vi "Periodic Tasks.vi"(8 "error in":errorcluster) -> ()   [LabVIEW 2019]
doc: "This VI runs in parallel to other tasks. It can contain as many user-defined periodic loops as you need. These can carry out PID or other sorts of timed response."
uses:
  <vilib>/Rock Robotics/WPI/ThirdParty/Phoenix-LabVIEW/Motor Controller/Controls/CTRE_Phoenix_MotorControl_ControlMode.ctl
  Control 1.ctl
  <vilib>/Rock Robotics/WPI/Solenoid/WPI_SolenoidValue.ctl
  <vilib>/Rock Robotics/WPI/ThirdParty/Phoenix-LabVIEW/Motor Controller/Get/CTRE_Phoenix_MotorController_GetSelectedSensorData.vi
  <vilib>/Rock Robotics/WPI/ThirdParty/Phoenix-LabVIEW/Motor Controller/Get/CTRE_Phoenix_MotorController_IntegratedSensorData_TalonFX.vi
  <vilib>/Rock Robotics/WPI/ThirdParty/Phoenix-LabVIEW/Motor Controller/Get/CTRE_Phoenix_MotorController_GetLimitSwitchStates.vi
  <vilib>/Rock Robotics/WPI/Solenoid/WPI_SolenoidSetEnum.vi
  <vilib>/Rock Robotics/WPI/RobotDrive/WPI_RobotDriveArcadeDrive_Standard(NoSaturation).vi
  <vilib>/Rock Robotics/WPI/ThirdParty/Phoenix-LabVIEW/Motor Controller/Get/CTRE_Phoenix_MotorController_GetQuadratureData.vi
  Talon SRX State Machine Enum.ctl
panel:
  in  "D":dbl
  in  "I":dbl
  in  "P":dbl=1.5
  in  "D 6":dbl
  in  "I 6":dbl
  in  "P 6":dbl=1.6
  in  "D 5":dbl
  in  "I 5":dbl
  in  "P 5":dbl=1.6
  out "Chicken 500 Low Home":bool
  out "Position":dbl format="%.2f"
  out "Dial":dbl(knob)=26.0 scale=26.0..156.0
  out "Degrees":dbl
  in  "D 2":dbl
  in  "I 2":dbl
  in  "P 2":dbl=1.6
  out "Low Home":bool
  out "Quadrature Position 2":i32
  # "90"
  # "45"
  # "F 90"
  # "F 45"
  # "Home"
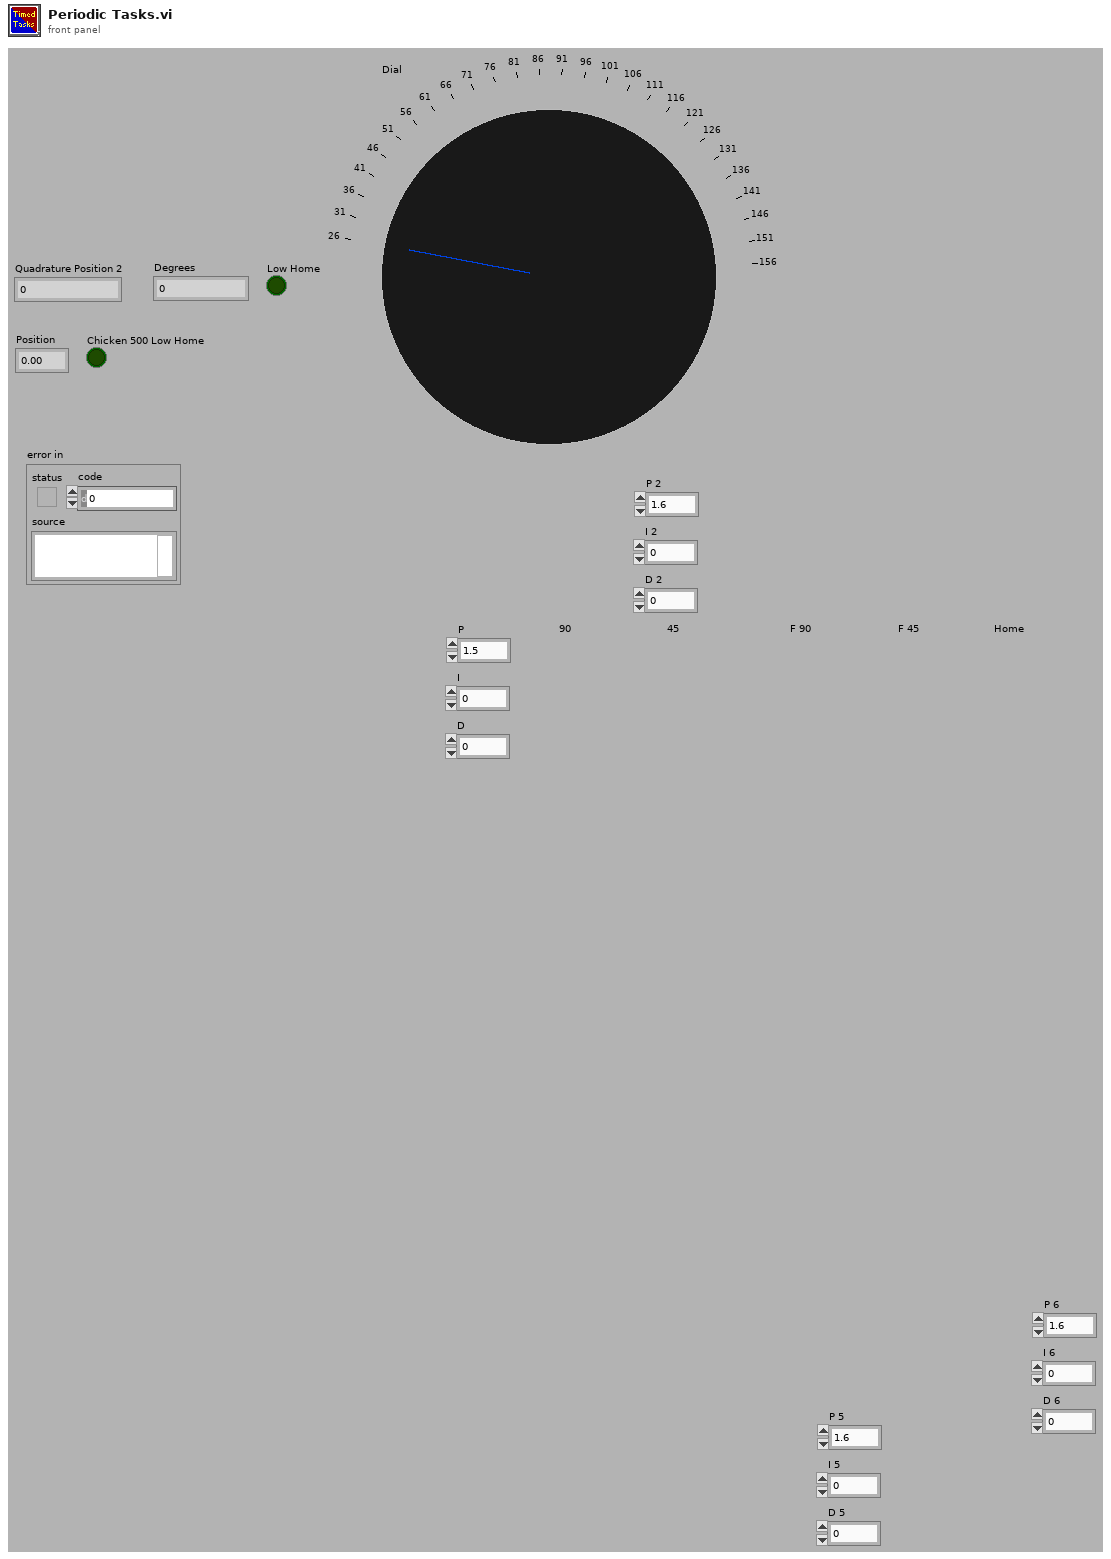
[diagram p1: front panel]
types:
  T1 = typedef "Talon SRX State Machine Enum.ctl" = enum16{"Wait", "Move 0", "Move 1", "Move 2", "Init"}
  T2 = typedef "Control 1.ctl" = enum16{"Wait", "F Move 0", "F Move 1", "F Move 2"}
  T3 = typedef "WPI_JoystickDevRef.ctl" = cluster{"Device":T4}
  T4 = typedef "WPI_JoystickDeviceEnum.ctl" = enum16{"USB 0", "USB 1", "USB 2", "USB 3", "USB 4", "USB 5"}
  T5 = typedef "WPI_MotorControlDeviceRef.ctl" = cluster{"DeviceStatus":errorcluster, "Type":T6, "PWM":cluster{"PWM Channel":T7, "DeadBand":T8}, "CAN":cluster{"Device Number":u8, "SetOutput VI Ref":variant, "GetOutput VI Ref":variant, "Enable VI Ref":variant, "Disable VI Ref":variant, "Data":variant}, "Invert":bool, "DIO PWM":cluster{"PWM \"Enable\" Channel":T7, "DIOChannel":T9, "PWM Rate":dbl}}
  T6 = typedef "WPI_MotorControlType.ctl" = enum16{"PWM", "CAN", "DIO PWM"}
  T7 = typedef "FPGA_DIOPWMChannel.ctl" = enum8{"PWM 0", "PWM 1", "PWM 2", "PWM 3", "PWM 4", "PWM 5", "PWM 6", "PWM 7", "PWM 8", "PWM 9", "PWM MXP 0", "PWM MXP 1", "PWM MXP 2", "PWM MXP 3", "PWM MXP 4", "PWM MXP 5", "PWM MXP 6", "PWM MXP 7", "PWM MXP 8", "PWM MXP 9", "Invalid"}
  T8 = typedef "WPI_PWMDeadband.ctl" = cluster{"Name":string, "maxPositivePwm":i32, "minPositivePwm":i32, "centerPwm":i32, "maxNegativePwm":i32, "minNegativePwm":i32, "angularRange":u16}
  T9 = typedef "FPGA_DIOChannel.ctl" = enum8{"DIO 0", "DIO 1", "DIO 2", "DIO 3", "DIO 4", "DIO 5", "DIO 6", "DIO 7", "DIO 8", "DIO 9", "DIO MXP 0", "DIO MXP 1", "DIO MXP 2", "DIO MXP 3", "DIO MXP 4", "DIO MXP 5", "DIO MXP 6", "DIO MXP 7", "DIO MXP 8", "DIO MXP 9", "DIO MXP 10", "DIO MXP 11", "DIO MXP 12", "DIO MXP 13", "DIO MXP 14", "DIO MXP 15", "SPI Port CS1", "SPI Port CS2", "SPI Port CS3", "SPI Port MISO", "SPI Port MOSI", "Invalid"}
  T10 = typedef "CTRE_Phoenix_MotorControl_ControlMode.ctl" = u16
  T11 = typedef "WPI_DigitalInputDevRef.ctl" = cluster{"DevStatus":errorcluster, "DIO Channel":T9}
  T12 = typedef "WPI_SolenoidValue.ctl" = enum16{"Off", "On", "Forward", "Reverse"}
  T13 = typedef "WPI_RobotDriveDevRef.ctl" = cluster{"DevStatus":errorcluster, "Motors[]":T5[], "Square Inputs":bool, "Max Output":dbl}
  T14 = typedef "WPI_SolenoidDevRef.ctl" = cluster{"DevStatus":errorcluster, "Pneumatics Control Module":u8, "Forward Solenoid Channel":T15, "Reverse Solenoid Channel":T15}
  T15 = typedef "WPI_SolenoidChannel.ctl" = enum8{"Solenoid 0", "Solenoid 1", "Solenoid 2", "Solenoid 3", "Solenoid 4", "Solenoid 5", "Solenoid 6", "Solenoid 7", "Invalid"}
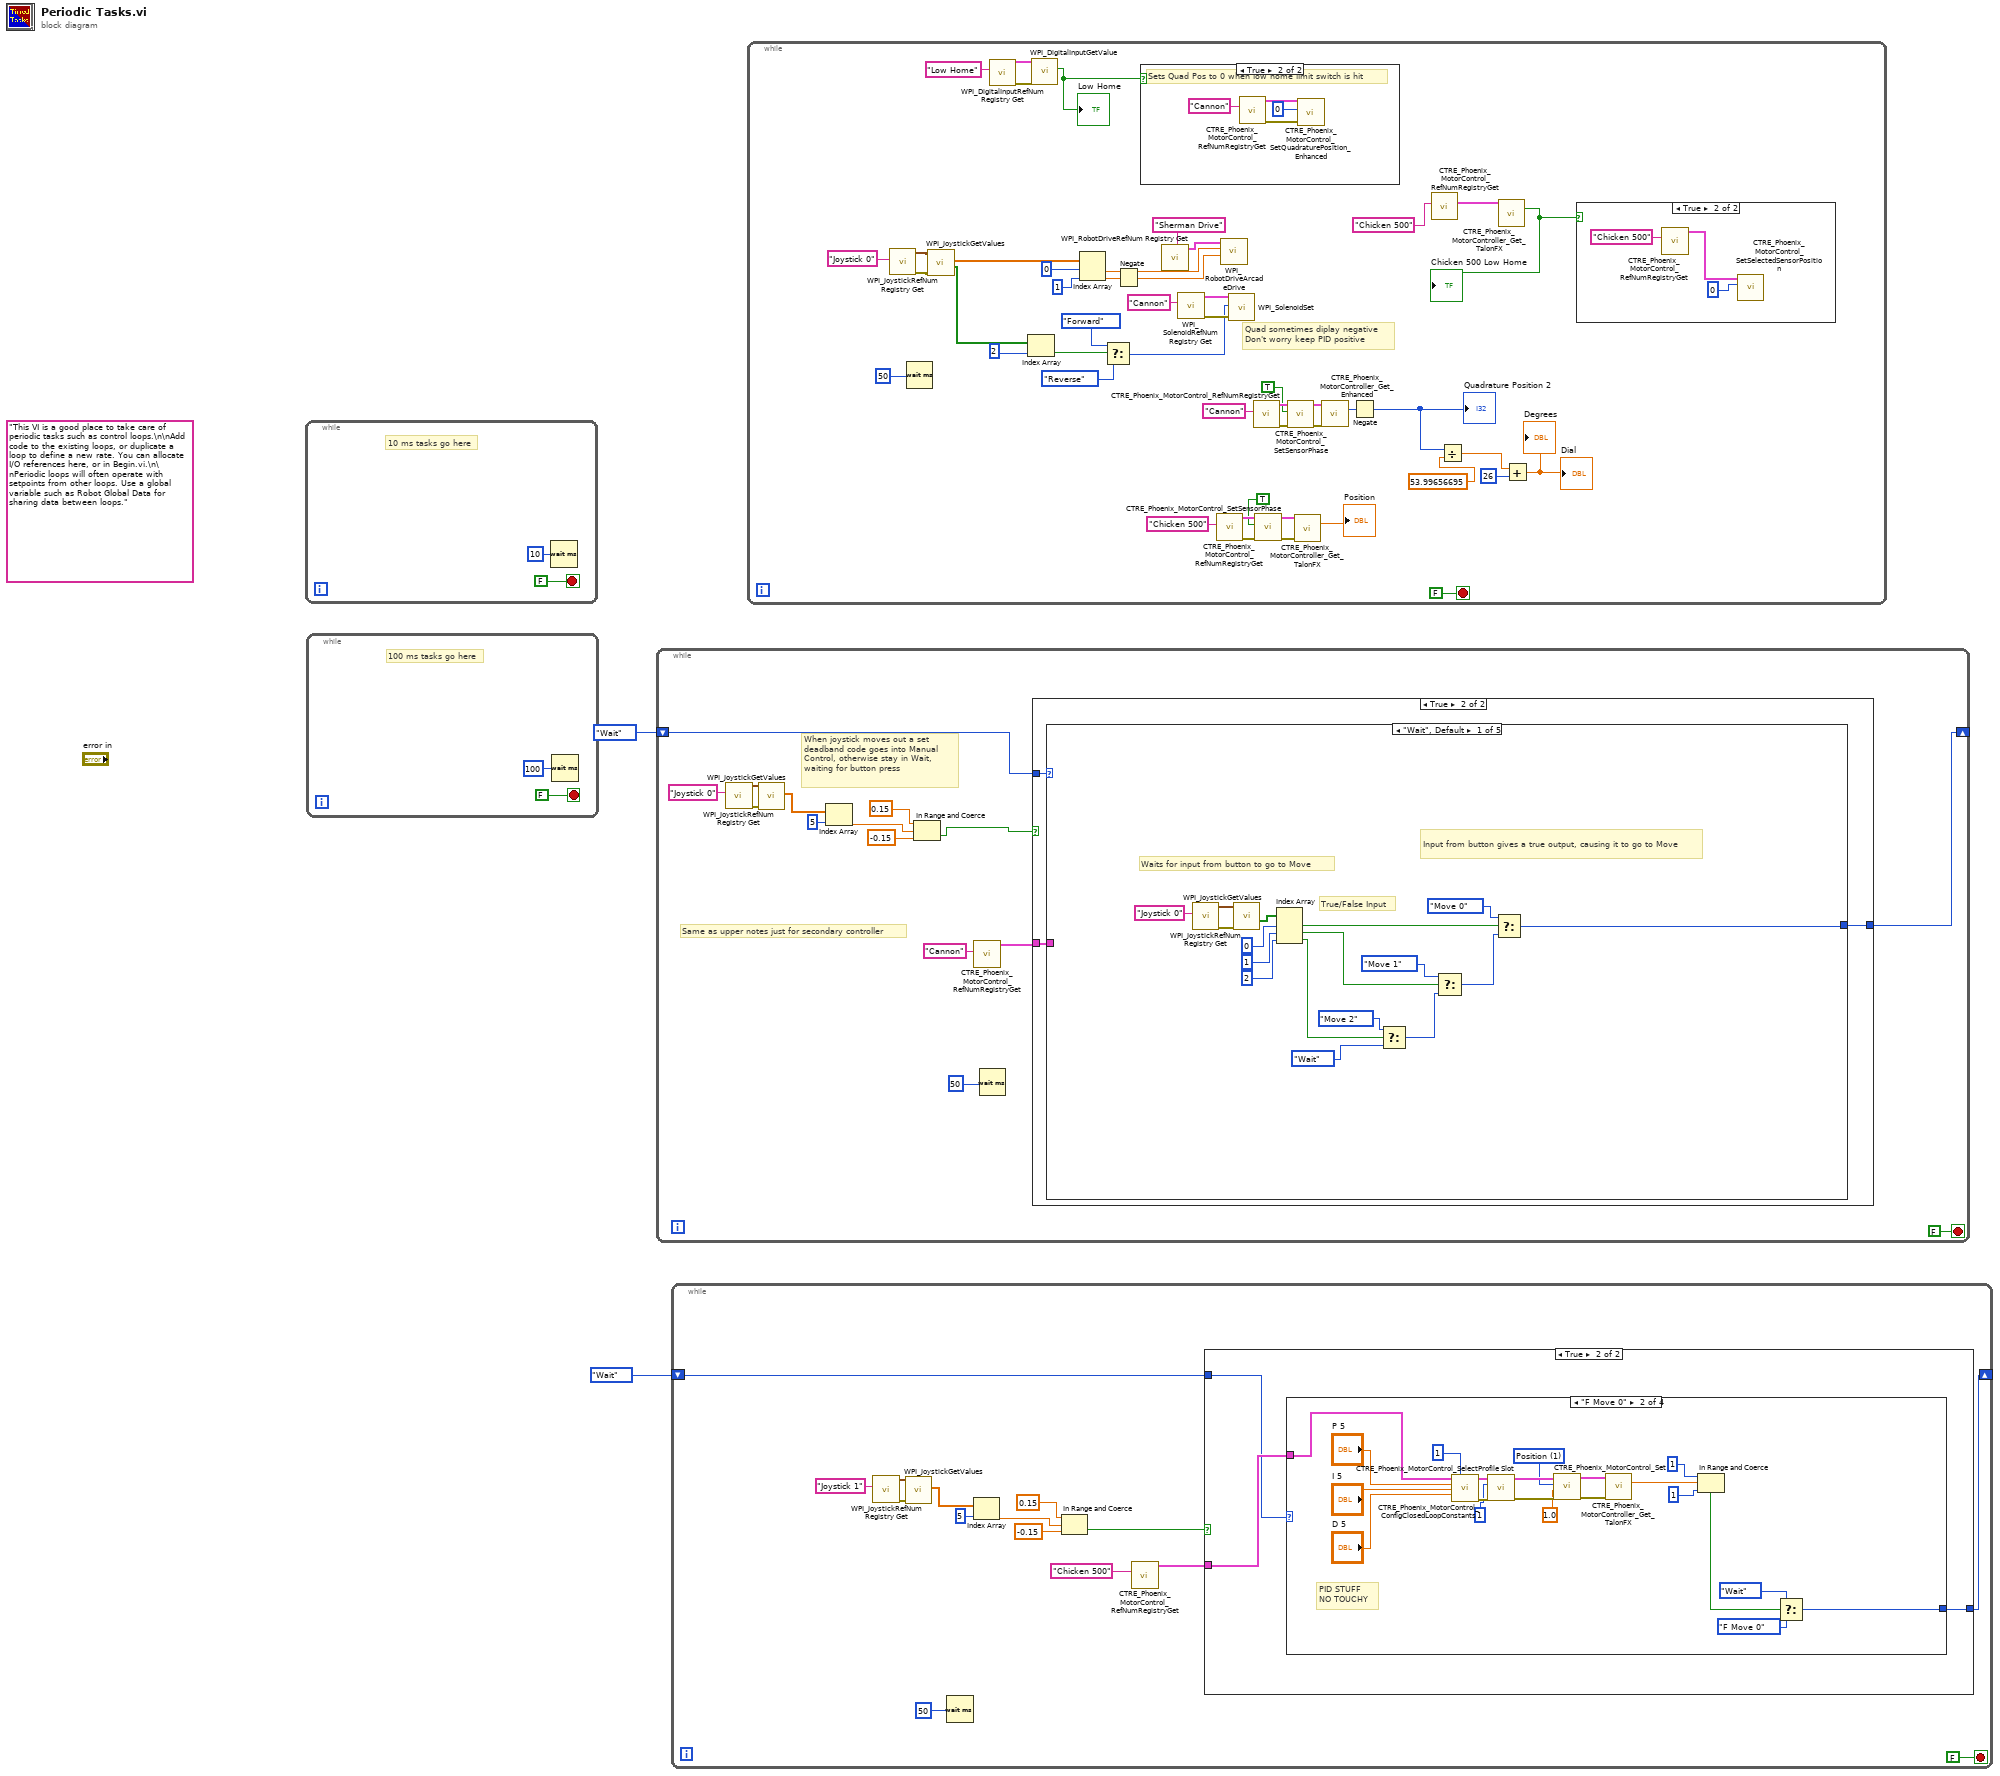
[diagram p0: block diagram]
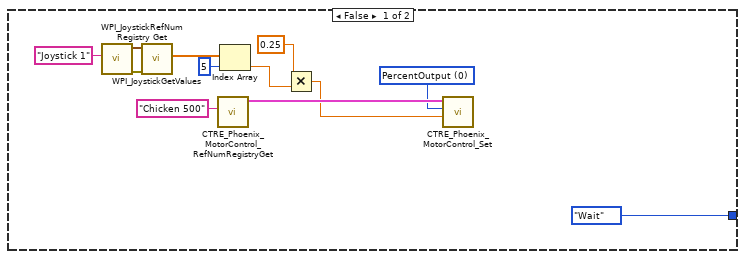
[diagram p2: hidden frame]
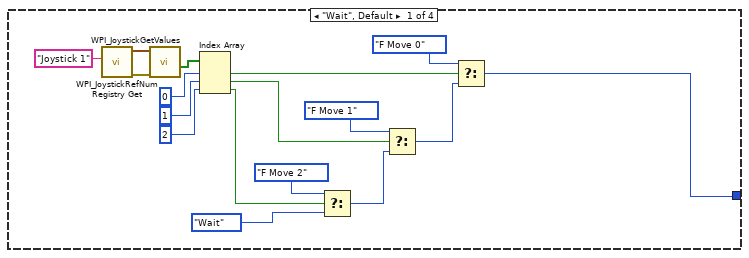
[diagram p3: hidden frame]
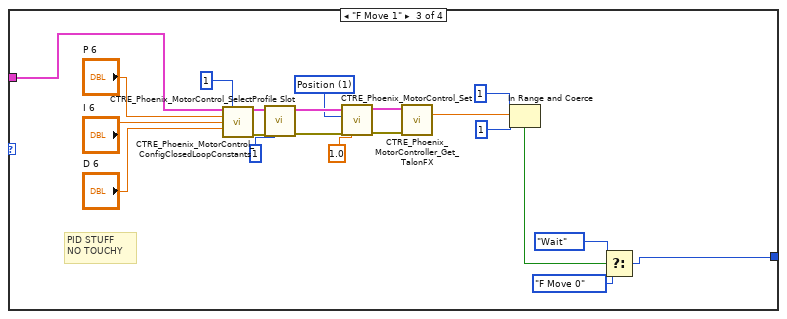
[diagram p4: hidden frame]
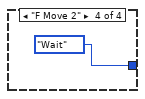
[diagram p5: hidden frame]
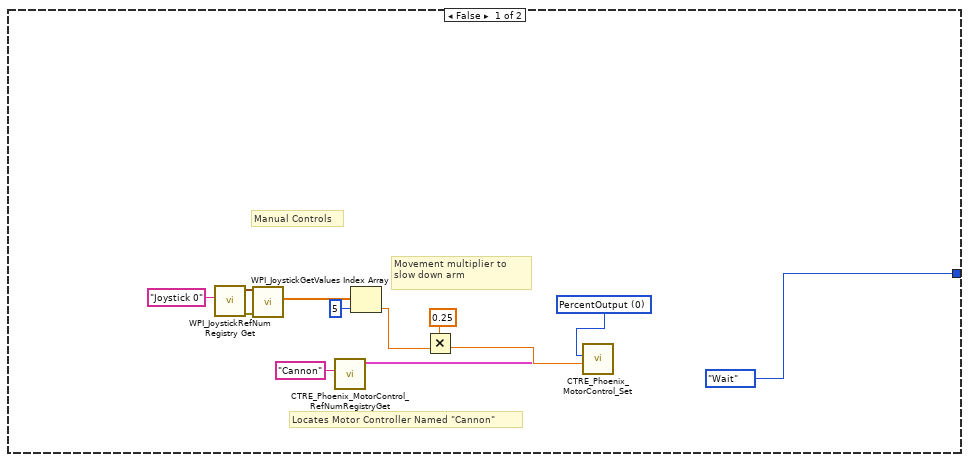
[diagram p8: hidden frame]
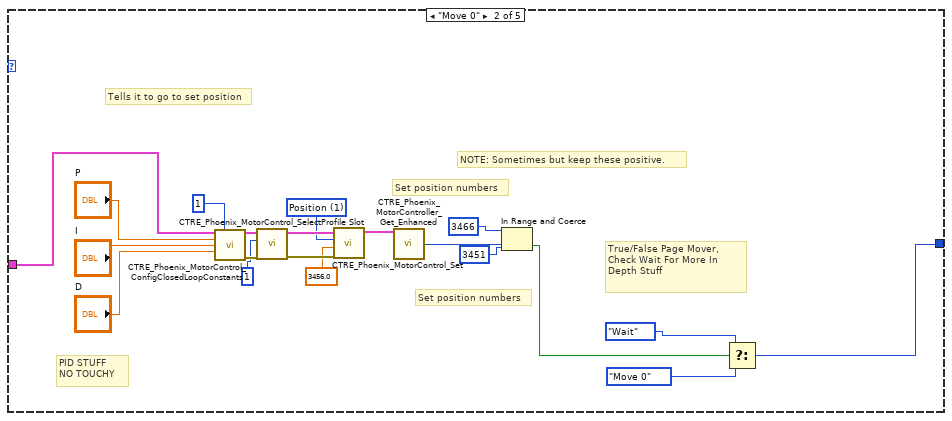
[diagram p9: hidden frame]
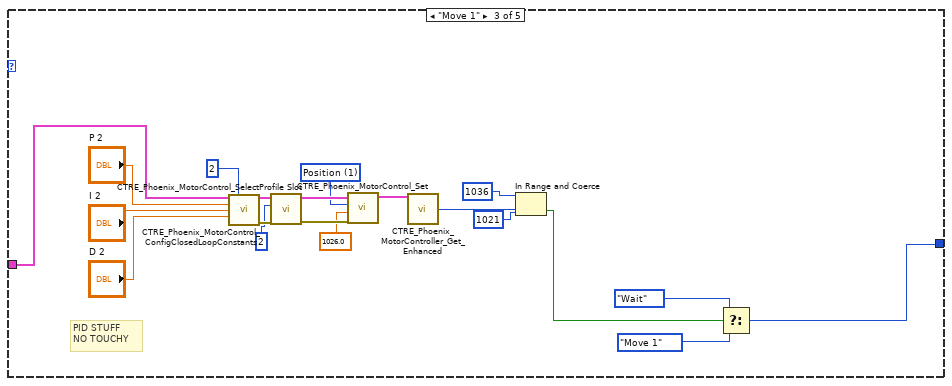
[diagram p10: hidden frame]
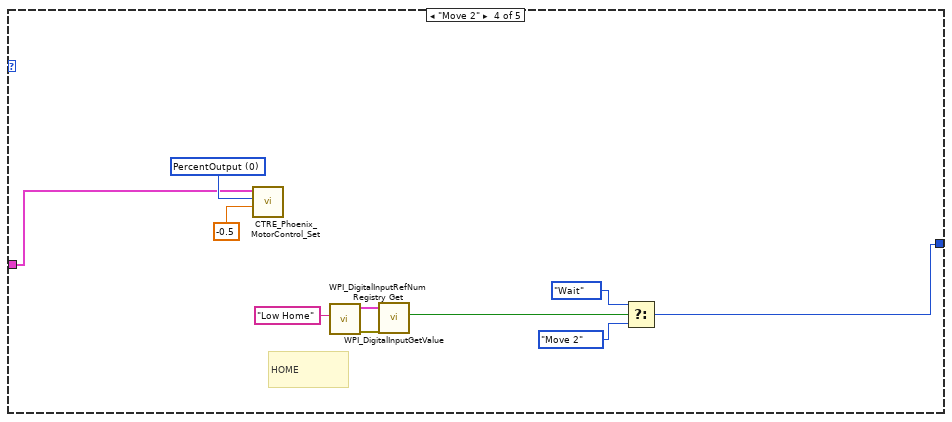
[diagram p11: hidden frame]
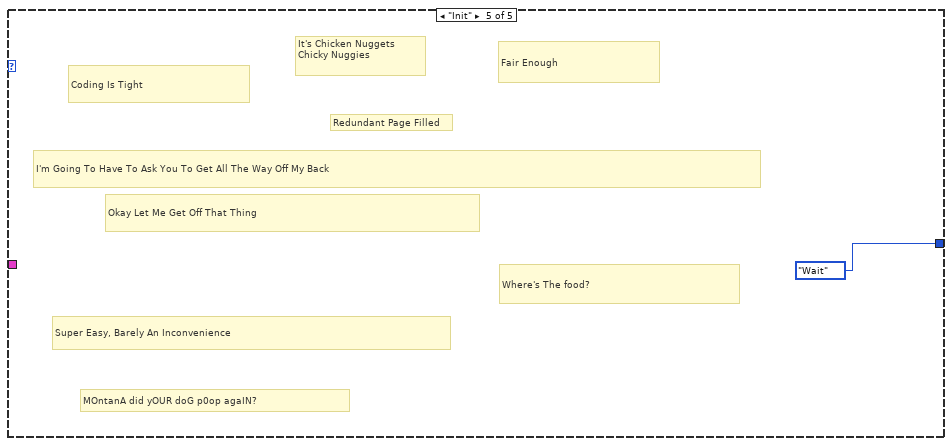
[diagram p12: hidden frame]
diagram:
  (unwired) "This VI is a good place to take care of periodic tasks such as control loops.\n\nAdd code to the existing loops, or duplicate a loop to define a new rate. You can allocate I/O references here, or in Begin.vi.\n\nPeriodic loops will often operate with setpoints from other loops. Use a global variable such as Robot Global Data for sharing data between loops."
  n1 = while {
    stop <- FALSE stop-if-true
    # "10 ms tasks go here"
    n2 = Wait (ms)(milliseconds to wait=u32 10) -> ()  [unwired: 1 out]
  }
  n3 = while {
    stop <- FALSE stop-if-true
    # "100 ms tasks go here"
    n4 = Wait (ms)(milliseconds to wait=u32 100) -> ()  [unwired: 1 out]
  }
  n5 = while {
    shift-right: [w7] -> _
    shift-left: Talon_SRX_State_Machine_Enum."Wait" -> [w21]
    stop <- FALSE stop-if-true
    # "Same as upper notes just for secondary controller"
    # "When joystick moves out a set deadband code goes into Manual Control, otherwise stay in Wait, waiting for button press"
    n6 = call <vilib>:"WPI_JoystickRefNum Registry Get.vi"("refnum name"="Joystick 0") -> ("error out"=w19:errorcluster, "JoystickDevRef"=w11:T3)  [unwired: 9 in]
    n7 = call <vilib>:"WPI_JoystickGetValues.vi"("error in (no error)"=w19, "JoystickDevRef"=w11) -> ("Axes"=w18:dbl[])  [unwired: 5 in, 4 out]
    n8 = Index Array(array=w18, index=5) -> (element=w17:dbl)
    n9 = In Range and Coerce(upper limit=0.15, x=w17, lower limit=-0.15) -> (In Range?=w8:bool)  [unwired: 1 out]
    n10 = call <vilib>:"CTRE_Phoenix_MotorControl_RefNumRegistryGet.vi"("refnum name"="Cannon") -> ("PhoenixMotorControlDevRef"=w10:T5)  [unwired: 9 in, 1 out]
    n11 = Wait (ms)(milliseconds to wait=50) -> ()  [unwired: 1 out]
    n12 = case shown="True" w8 {
      tunnel: w21 -> [_ w36]
      tunnel: w10 -> [_ w35]
      tunnel: [Talon_SRX_State_Machine_Enum."Wait" w34] -> w7
      frame False {
        w23 = T10 0 items=["PercentOutput"=0, "Position"=1, "Velocity"=2, "Current"=3, "Follower"=5, "MotionProfile"=6, "MotionMagic"=7, "MotionProfileArc"=10, "Disabled"=15] ("Control Mode")
        # "Locates Motor Controller Named \"Cannon\""
        # "Movement multiplier to slow down arm"
        # "Manual Controls"
        n13 = call <vilib>:"WPI_JoystickRefNum Registry Get.vi"("refnum name"="Joystick 0") -> ("error out"=w31:errorcluster, "JoystickDevRef"=w32:T3)  [unwired: 9 in]
        n14 = call <vilib>:"WPI_JoystickGetValues.vi"("error in (no error)"=w31, "JoystickDevRef"=w32) -> ("Axes"=w30:dbl[])  [unwired: 5 in, 4 out]
        n15 = call <vilib>:"CTRE_Phoenix_MotorControl_RefNumRegistryGet.vi"("refnum name"="Cannon") -> ("PhoenixMotorControlDevRef"=w24:T5)  [unwired: 9 in, 1 out]
        n16 = Index Array(array=w30, index=5) -> (element=w28:dbl)
        n17 = Multiply(x=0.25, y=w28) -> (x*y=w25:dbl)
        n18 = call <vilib>:"CTRE_Phoenix_MotorControl_Set.vi"("Output"=w25, "Control Mode"=w23, "PhoenixMotorControlDevRef"=w24) -> ()  [unwired: 7 in, 2 out]
      }
      frame True {
        n19 = case shown="\"Wait\", Default" w36 {
          tunnel: w35 -> [_ w54 w77 w94 _]
          tunnel: [w37 w55 w74 w97 Talon_SRX_State_Machine_Enum."Wait"] -> w34
          frame "Wait", Default {
            # "True/False Input"
            # "Input from button gives a true output, causing it to go to Move"
            # "Waits for input from button to go to Move"
            n20 = call <vilib>:"WPI_JoystickRefNum Registry Get.vi"("refnum name"="Joystick 0") -> ("error out"=w53:errorcluster, "JoystickDevRef"=w52:T3)  [unwired: 9 in]
            n21 = call <vilib>:"WPI_JoystickGetValues.vi"("error in (no error)"=w53, "JoystickDevRef"=w52) -> ("Buttons"=w50:bool[])  [unwired: 5 in, 4 out]
            n22 = Index Array(array=w50, index #1=0 ("index"), index #2=1 ("index"), index #3=2 ("index")) -> (element #1=w48:bool, element #2=w46:bool, element #3=w42:bool)
            n23 = Select(t=Talon_SRX_State_Machine_Enum."Move 2", s=w42, f=Talon_SRX_State_Machine_Enum."Wait") -> (s? t:f=w43:T1)
            n24 = Select(t=Talon_SRX_State_Machine_Enum."Move 1", s=w46, f=w43) -> (s? t:f=w45:T1)
            n25 = Select(t=Talon_SRX_State_Machine_Enum."Move 0", s=w48, f=w45) -> (s? t:f=w37:T1)
          }
          frame "Move 0" {
            w61 = T10 1 items=["PercentOutput"=0, "Position"=1, "Velocity"=2, "Current"=3, "Follower"=5, "MotionProfile"=6, "MotionMagic"=7, "MotionProfileArc"=10, "Disabled"=15] ("Control Mode")
            # "Tells it to go to set position"
            # "NOTE: Sometimes but keep these positive."
            # "PID STUFF\nNO TOUCHY"
            # "True/False Page Mover, Check Wait For More In Depth Stuff"
            # "Set position numbers"
            # "Set position numbers"
            n26 = call <vilib>:"CTRE_Phoenix_MotorControl_ConfigClosedLoopConstants.vi"("PhoenixMotorControlDevRef"=w54, "slotIdx"=1, "P"="P", "I"="I", "D"="D") -> ("PhoenixMotorControlDevRef"=w68:T5, "error out"=w69:errorcluster)  [unwired: 9 in]
            n27 = call <vilib>:"CTRE_Phoenix_MotorControl_SelectProfile Slot.vi"("error in (no error)"=w69, "slotIdx"=1, "PhoenixMotorControlDevRef"=w68) -> ("error out"=w70:errorcluster, "PhoenixMotorControlDevRef"=w71:T5)  [unwired: 7 in]
            n28 = call <vilib>:"CTRE_Phoenix_MotorControl_Set.vi"("error in (no error)"=w70, "Output"=3456.0, "Control Mode"=w61, "PhoenixMotorControlDevRef"=w71) -> ("PhoenixMotorControlDevRef"=w72:T5)  [unwired: 6 in, 1 out]
            n29 = call-poly <vilib>:"CTRE_Phoenix_MotorController_Get_Enhanced.vi"("PhoenixMotorControlDevRef"=w72) -> ("Velocity (Raw Sensor Units per 100 ms)"=w73:i32)  [unwired: 11 in, 3 out]
            n30 = In Range and Coerce(upper limit=3466, x=w73, lower limit=3451) -> (In Range?=w58:bool)  [unwired: 1 out]
            n31 = Select(t=Talon_SRX_State_Machine_Enum."Wait", s=w58, f=Talon_SRX_State_Machine_Enum."Move 0") -> (s? t:f=w55:T1)
          }
          frame "Move 1" {
            w81 = T10 1 items=["PercentOutput"=0, "Position"=1, "Velocity"=2, "Current"=3, "Follower"=5, "MotionProfile"=6, "MotionMagic"=7, "MotionProfileArc"=10, "Disabled"=15] ("Control Mode")
            # "PID STUFF\nNO TOUCHY"
            n32 = call <vilib>:"CTRE_Phoenix_MotorControl_ConfigClosedLoopConstants.vi"("PhoenixMotorControlDevRef"=w77, "slotIdx"=2, "P"="P 2", "I"="I 2", "D"="D 2") -> ("PhoenixMotorControlDevRef"=w88:T5, "error out"=w89:errorcluster)  [unwired: 9 in]
            n33 = call <vilib>:"CTRE_Phoenix_MotorControl_SelectProfile Slot.vi"("error in (no error)"=w89, "slotIdx"=2, "PhoenixMotorControlDevRef"=w88) -> ("error out"=w90:errorcluster, "PhoenixMotorControlDevRef"=w91:T5)  [unwired: 7 in]
            n34 = call <vilib>:"CTRE_Phoenix_MotorControl_Set.vi"("error in (no error)"=w90, "Output"=1026.0, "Control Mode"=w81, "PhoenixMotorControlDevRef"=w91) -> ("PhoenixMotorControlDevRef"=w92:T5)  [unwired: 6 in, 1 out]
            n35 = call-poly <vilib>:"CTRE_Phoenix_MotorController_Get_Enhanced.vi"("PhoenixMotorControlDevRef"=w92) -> ("Velocity (Raw Sensor Units per 100 ms)"=w93:i32)  [unwired: 11 in, 3 out]
            n36 = In Range and Coerce(upper limit=1036, x=w93, lower limit=1021) -> (In Range?=w78:bool)  [unwired: 1 out]
            n37 = Select(t=Talon_SRX_State_Machine_Enum."Wait", s=w78, f=Talon_SRX_State_Machine_Enum."Move 1") -> (s? t:f=w74:T1)
          }
          frame "Move 2" {
            w102 = T10 0 items=["PercentOutput"=0, "Position"=1, "Velocity"=2, "Current"=3, "Follower"=5, "MotionProfile"=6, "MotionMagic"=7, "MotionProfileArc"=10, "Disabled"=15] ("Control Mode")
            # "HOME"
            n38 = call <vilib>:"CTRE_Phoenix_MotorControl_Set.vi"("Output"=-0.5, "Control Mode"=w102, "PhoenixMotorControlDevRef"=w94) -> ()  [unwired: 7 in, 2 out]
            n39 = call <vilib>:"WPI_DigitalInputRefNum Registry Get.vi"("refnum name"="Low Home") -> ("error out"=w101:errorcluster, "DigitalInputDevRef"=w98:T11)  [unwired: 9 in]
            n40 = call <vilib>:"WPI_DigitalInputGetValue.vi"("error in (no error)"=w101, "DigitalInputDevRef"=w98) -> ("Value"=w99:bool)  [unwired: 7 in, 2 out]
            n41 = Select(t=Talon_SRX_State_Machine_Enum."Wait", s=w99, f=Talon_SRX_State_Machine_Enum."Move 2") -> (s? t:f=w97:T1)
          }
          frame "Init" {
            # "MOntanA did yOUR doG p0op agaIN?"
            # "It's Chicken Nuggets\nChicky Nuggies"
            # "Where's The food?"
            # "Redundant Page Filled"
            # "Okay Let Me Get Off That Thing"
            # "I'm Going To Have To Ask You To Get All The Way Off My Back"
            # "Fair Enough"
            # "Coding Is Tight"
            # "Super Easy, Barely An Inconvenience"
          }
        }
      }
    }
  }
  n42 = while {
    shift-right: [w106] -> _
    shift-left: Control_1."Wait" -> [w107]
    stop <- FALSE stop-if-true
    n43 = call <vilib>:"WPI_JoystickRefNum Registry Get.vi"("refnum name"="Joystick 1") -> ("error out"=w116:errorcluster, "JoystickDevRef"=w119:T3)  [unwired: 9 in]
    n44 = call <vilib>:"WPI_JoystickGetValues.vi"("error in (no error)"=w116, "JoystickDevRef"=w119) -> ("Axes"=w117:dbl[])  [unwired: 5 in, 4 out]
    n45 = Wait (ms)(milliseconds to wait=50) -> ()  [unwired: 1 out]
    n46 = Index Array(array=w117, index=5) -> (element=w118:dbl)
    n47 = In Range and Coerce(upper limit=0.15, x=w118, lower limit=-0.15) -> (In Range?=w109:bool)  [unwired: 1 out]
    n48 = call <vilib>:"CTRE_Phoenix_MotorControl_RefNumRegistryGet.vi"("refnum name"="Chicken 500") -> ("PhoenixMotorControlDevRef"=w108:T5)  [unwired: 9 in, 1 out]
    n49 = case shown="True" w109 {
      tunnel: w108 -> [_ w134]
      tunnel: w107 -> [_ w133]
      tunnel: [Control_1."Wait" w132] -> w106
      frame False {
        w125 = T10 0 items=["PercentOutput"=0, "Position"=1, "Velocity"=2, "Current"=3, "Follower"=5, "MotionProfile"=6, "MotionMagic"=7, "MotionProfileArc"=10, "Disabled"=15] ("Control Mode")
        n50 = call <vilib>:"WPI_JoystickRefNum Registry Get.vi"("refnum name"="Joystick 1") -> ("error out"=w126:errorcluster, "JoystickDevRef"=w127:T3)  [unwired: 9 in]
        n51 = call <vilib>:"WPI_JoystickGetValues.vi"("error in (no error)"=w126, "JoystickDevRef"=w127) -> ("Axes"=w128:dbl[])  [unwired: 5 in, 4 out]
        n52 = call <vilib>:"CTRE_Phoenix_MotorControl_RefNumRegistryGet.vi"("refnum name"="Chicken 500") -> ("PhoenixMotorControlDevRef"=w131:T5)  [unwired: 9 in, 1 out]
        n53 = Index Array(array=w128, index=5) -> (element=w129:dbl)
        n54 = Multiply(x=0.25, y=w129) -> (x*y=w130:dbl)
        n55 = call <vilib>:"CTRE_Phoenix_MotorControl_Set.vi"("Output"=w130, "Control Mode"=w125, "PhoenixMotorControlDevRef"=w131) -> ()  [unwired: 7 in, 2 out]
      }
      frame True {
        n56 = case shown="\"F Move 0\"" w133 {
          tunnel: w134 -> [_ w153 w174 _]
          tunnel: [w139 w152 w173 Control_1."Wait"] -> w132
          frame "Wait", Default {
            n57 = call <vilib>:"WPI_JoystickRefNum Registry Get.vi"("refnum name"="Joystick 1") -> ("error out"=w151:errorcluster, "JoystickDevRef"=w150:T3)  [unwired: 9 in]
            n58 = call <vilib>:"WPI_JoystickGetValues.vi"("error in (no error)"=w151, "JoystickDevRef"=w150) -> ("Buttons"=w148:bool[])  [unwired: 5 in, 4 out]
            n59 = Index Array(array=w148, index #1=0 ("index"), index #2=1 ("index"), index #3=2 ("index")) -> (element #1=w146:bool, element #2=w144:bool, element #3=w140:bool)
            n60 = Select(t=Control_1."F Move 2", s=w140, f=Control_1."Wait") -> (s? t:f=w141:T2)
            n61 = Select(t=Control_1."F Move 1", s=w144, f=w141) -> (s? t:f=w143:T2)
            n62 = Select(t=Control_1."F Move 0", s=w146, f=w143) -> (s? t:f=w139:T2)
          }
          frame "F Move 0" {
            w162 = T10 1 items=["PercentOutput"=0, "Position"=1, "Velocity"=2, "Current"=3, "Follower"=5, "MotionProfile"=6, "MotionMagic"=7, "MotionProfileArc"=10, "Disabled"=15] ("Control Mode")
            # "PID STUFF\nNO TOUCHY"
            n63 = call <vilib>:"CTRE_Phoenix_MotorControl_ConfigClosedLoopConstants.vi"("PhoenixMotorControlDevRef"=w153, "slotIdx"=1, "P"="P 5", "I"="I 5", "D"="D 5") -> ("PhoenixMotorControlDevRef"=w169:T5, "error out"=w170:errorcluster)  [unwired: 9 in]
            n64 = call <vilib>:"CTRE_Phoenix_MotorControl_SelectProfile Slot.vi"("error in (no error)"=w170, "slotIdx"=1, "PhoenixMotorControlDevRef"=w169) -> ("error out"=w171:errorcluster, "PhoenixMotorControlDevRef"=w172:T5)  [unwired: 7 in]
            n65 = call <vilib>:"CTRE_Phoenix_MotorControl_Set.vi"("error in (no error)"=w171, "Output"=1.0, "Control Mode"=w162, "PhoenixMotorControlDevRef"=w172) -> ("error out"=w155:errorcluster, "PhoenixMotorControlDevRef"=w156:T5)  [unwired: 6 in]
            n66 = call-poly <vilib>:"CTRE_Phoenix_MotorController_Get_TalonFX.vi"("PhoenixMotorControlDevRef"=w156, "error in"=w155) -> ("Position"=w154:dbl)  [unwired: 9 in, 4 out]
            n67 = In Range and Coerce(upper limit=1, x=w154, lower limit=1) -> (In Range?=w159:bool)  [unwired: 1 out]
            n68 = Select(t=Control_1."Wait", s=w159, f=Control_1."F Move 0") -> (s? t:f=w152:T2)
          }
          frame "F Move 1" {
            w179 = T10 1 items=["PercentOutput"=0, "Position"=1, "Velocity"=2, "Current"=3, "Follower"=5, "MotionProfile"=6, "MotionMagic"=7, "MotionProfileArc"=10, "Disabled"=15] ("Control Mode")
            # "PID STUFF\nNO TOUCHY"
            n69 = call <vilib>:"CTRE_Phoenix_MotorControl_ConfigClosedLoopConstants.vi"("PhoenixMotorControlDevRef"=w174, "slotIdx"=1, "P"="P 6", "I"="I 6", "D"="D 6") -> ("PhoenixMotorControlDevRef"=w186:T5, "error out"=w185:errorcluster)  [unwired: 9 in]
            n70 = call <vilib>:"CTRE_Phoenix_MotorControl_SelectProfile Slot.vi"("error in (no error)"=w185, "slotIdx"=1, "PhoenixMotorControlDevRef"=w186) -> ("error out"=w184:errorcluster, "PhoenixMotorControlDevRef"=w183:T5)  [unwired: 7 in]
            n71 = call <vilib>:"CTRE_Phoenix_MotorControl_Set.vi"("error in (no error)"=w184, "Output"=1.0, "Control Mode"=w179, "PhoenixMotorControlDevRef"=w183) -> ("error out"=w192:errorcluster, "PhoenixMotorControlDevRef"=w191:T5)  [unwired: 6 in]
            n72 = call-poly <vilib>:"CTRE_Phoenix_MotorController_Get_TalonFX.vi"("PhoenixMotorControlDevRef"=w191, "error in"=w192) -> ("Position"=w193:dbl)  [unwired: 9 in, 4 out]
            n73 = In Range and Coerce(upper limit=1, x=w193, lower limit=1) -> (In Range?=w190:bool)  [unwired: 1 out]
            n74 = Select(t=Control_1."Wait", s=w190, f=Control_1."F Move 0") -> (s? t:f=w173:T2)
          }
          frame "F Move 2" {
          }
        }
      }
    }
  }
  n75 = while {
    stop <- FALSE stop-if-true
    # "Quad sometimes diplay negative\nDon't worry keep PID positive"
    n76 = call <vilib>:"WPI_JoystickRefNum Registry Get.vi"("refnum name"="Joystick 0") -> ("error out"=w237:errorcluster, "JoystickDevRef"=w236:T3)  [unwired: 9 in]
    n77 = Wait (ms)(milliseconds to wait=50) -> ()  [unwired: 1 out]
    n78 = call <vilib>:"WPI_JoystickGetValues.vi"("error in (no error)"=w237, "JoystickDevRef"=w236) -> ("Buttons"=w233:bool[], "Axes"=w234:dbl[])  [unwired: 5 in, 3 out]
    n79 = call <vilib>:"WPI_DigitalInputRefNum Registry Get.vi"("refnum name"="Low Home") -> ("error out"=w241:errorcluster, "DigitalInputDevRef"=w240:T11)  [unwired: 9 in]
    n80 = Index Array(array=w233, index=2) -> (element=w231:bool)
    n81 = call <vilib>:"WPI_DigitalInputGetValue.vi"("error in (no error)"=w241, "DigitalInputDevRef"=w240) -> ("Value"=w238:bool)  [unwired: 7 in, 2 out]
    "Low Home" <- w238
    n82 = Index Array(array=w234, index #1=0 ("index"), index #2=1 ("index")) -> (element #1=w218:dbl, element #2=w220:dbl)
    n83 = Select(t=WPI_SolenoidValue."Forward" ("Value"), s=w231, f=WPI_SolenoidValue."Reverse" ("Value")) -> (s? t:f=w226:T12)
    n84 = Negate(x=w220) -> (-x=w219:dbl)
    n85 = case shown="True" w238 {
      frame False {
      }
      frame True {
        # "Sets Quad Pos to 0 when low home limit switch is hit"
        n86 = call <vilib>:"CTRE_Phoenix_MotorControl_RefNumRegistryGet.vi"("refnum name"="Cannon") -> ("error out"=w246:errorcluster, "PhoenixMotorControlDevRef"=w245:T5)  [unwired: 9 in]
        n87 = call <vilib>:"CTRE_Phoenix_MotorControl_SetQuadraturePosition_Enhanced.vi"("error in (no error)"=w246, "New Position"=0, "PhoenixMotorControlDevRef"=w245) -> ()  [unwired: 7 in, 2 out]
      }
    }
    n88 = call <vilib>:"WPI_RobotDriveRefNum Registry Get.vi"("refnum name"="Sherman Drive") -> ("RobotDriveDevRef"=w222:T13)  [unwired: 9 in, 1 out]
    n89 = call <vilib>:"WPI_SolenoidRefNum Registry Get.vi"("refnum name"="Cannon") -> ("error out"=w230:errorcluster, "SolenoidDevRef"=w229:T14)  [unwired: 9 in]
    n90 = call <vilib>:"CTRE_Phoenix_MotorControl_RefNumRegistryGet.vi"("refnum name"="Chicken 500") -> ("error out"=w203:errorcluster, "PhoenixMotorControlDevRef"=w204:T5)  [unwired: 9 in]
    n91 = call-poly <vilib>:"WPI_RobotDriveArcadeDrive.vi"("Y axis value"=w219, "X axis value"=w218, "RobotDriveDevRef"=w222) -> ()  [unwired: 6 in, 3 out]
    n92 = call-poly <vilib>:"WPI_SolenoidSet.vi"("error in (no error)"=w230, "Value"=w226, "SolenoidDevRef"=w229) -> ()  [unwired: 7 in, 2 out]
    n93 = call <vilib>:"CTRE_Phoenix_MotorControl_RefNumRegistryGet.vi"("refnum name"="Cannon") -> ("error out"=w216:errorcluster, "PhoenixMotorControlDevRef"=w217:T5)  [unwired: 9 in]
    n94 = call <vilib>:"CTRE_Phoenix_MotorControl_SetSensorPhase.vi"("error in (no error)"=w203, "PhaseSensor"=TRUE, "PhoenixMotorControlDevRef"=w204) -> ("error out"=w199:errorcluster, "PhoenixMotorControlDevRef"=w200:T5)  [unwired: 7 in]
    n95 = call <vilib>:"CTRE_Phoenix_MotorControl_SetSensorPhase.vi"("PhaseSensor"=TRUE, "PhoenixMotorControlDevRef"=w217) -> ("PhoenixMotorControlDevRef"=w211:T5)  [unwired: 8 in, 1 out]
    n96 = call-poly <vilib>:"CTRE_Phoenix_MotorController_Get_TalonFX.vi"("PhoenixMotorControlDevRef"=w200, "error in"=w199) -> ("Position"=→"Position":dbl)  [unwired: 9 in, 4 out]
    n97 = call-poly <vilib>:"CTRE_Phoenix_MotorController_Get_Enhanced.vi"("PhoenixMotorControlDevRef"=w211, "error in"=w216) -> ("Quadrature Position"=w215:i32)  [unwired: 10 in, 3 out]
    n98 = Negate(x=w215) -> (-x=w205:i32)
    "Quadrature Position 2" <- w205
    n99 = call <vilib>:"CTRE_Phoenix_MotorControl_RefNumRegistryGet.vi"("refnum name"="Chicken 500") -> ("PhoenixMotorControlDevRef"=w195:T5)  [unwired: 9 in, 1 out]
    n100 = Divide(x=w205, y=53.99656695) -> (x/y=w207:dbl)
    n101 = call-poly <vilib>:"CTRE_Phoenix_MotorController_Get_TalonFX.vi"("PhoenixMotorControlDevRef"=w195) -> ("Forward Limit Closed?"=w197:bool)  [unwired: 11 in, 3 out]
    "Chicken 500 Low Home" <- w197
    n102 = Add(x=w207, y=26) -> (x+y=→"Degrees" →"Dial":dbl)
    n103 = case shown="True" w197 {
      frame False {
      }
      frame True {
        n104 = call <vilib>:"CTRE_Phoenix_MotorControl_RefNumRegistryGet.vi"("refnum name"="Chicken 500") -> ("PhoenixMotorControlDevRef"=w242:T5)  [unwired: 9 in, 1 out]
        n105 = call <vilib>:"CTRE_Phoenix_MotorControl_SetSelectedSensorPosition.vi"("New Sensor Position"=0, "PhoenixMotorControlDevRef"=w242) -> ()  [unwired: 8 in, 2 out]
      }
    }
  }
